vi "Slow Axis Waveform Generator.vi"(4 "Flyback Lines":u16, 5 "Number Data of Points":i32, 6 "Scan Parameters":T1, 7 "Image Acquisition Parameters":T2={"Scan Type"=enum."Sample Scanning", "Scan Mode"=enum."XY", "Fast Axis Frequency (Hz)"=100.0, "Image Format"=128, "Line Accumulations"=1, "Frames Per Capture"=1, "Frames Accumulations"=1, "Image Dimension (um)"=[], "Number of Z Steps"=1, "Z Steps Size (um)"=1.0, "Pixel Size (nm)"=[]} {"Z Steps Size (um)" min=0.0; "Number of Z Steps" min=1; "Frames Accumulations" min=1; "Frames Per Capture" min=1; "Line Accumulations" min=1; "Image Format" items=["64 x 64"=64, "128 x 128"=128, "256 x 256"=256, "512 x 512"=512, "1024 x 1024"=1024, "2048 x 2048"=2048]}) -> (0 "Linear Ramp End":u32, 1 "Slow Axis Frequency":dbl, 2 "Slow Axis Waveform":dbl[](array[numeric]), 3 "Flyback Lines":u16)   [LabVIEW 2016]
uses:
  Type Defs/Image Acquisition Parameters.ctl
  Scan Parameters.ctl
panel:
  out "XY Graph":cluster{"y":dbl[], "t":dbl[]}(graph)
  # "Copyright (C) 2020 Edward S Allgeyer\n\nRedistribution and use in source and binary forms, with or without\nmodification, are permitted provided that the following conditions\nare met:\n\n1. Redistributions of source code must retain the above copyright\n   notice, this list of conditions and the following disclaimer.\n\n2. Redistributions in binary form must reproduce the above copyright\n   notice, this list of conditions and the following disclaimer in\n   the documentation and/or other materials provided with the\n   distribution.\n\n3. Neither the name of the copyright holder nor the names of its\n   contributors may be used to endorse or promote products derived\n   from this software without specific prior written permission.\n\nTHIS SOFTWARE IS PROVIDED BY THE COPYRIGHT HOLDERS AND CONTRIBUTORS\n\"AS IS\" AND ANY EXPRESS OR IMPLIED WARRANTIES, INCLUDING, BUT NOT\nLIMITED TO, THE IMPLIED WARRANTIES OF MERCHANTABILITY AND FITNESS\nFOR A PARTICULAR PURPOSE ARE DISCLAIMED. IN NO EVENT SHALL THE\nCOPYRIGHT HOLDER OR CONTRIBUTORS BE LIABLE FOR ANY DIRECT, INDIRECT,\nINCIDENTAL, SPECIAL, EXEMPLARY, OR CONSEQUENTIAL DAMAGES (INCLUDING,\nBUT NOT LIMITED TO, PROCUREMENT OF SUBSTITUTE GOODS OR SERVICES;\nLOSS OF USE, DATA, OR PROFITS; OR BUSINESS INTERRUPTION) HOWEVER\nCAUSED AND ON ANY THEORY OF LIABILITY, WHETHER IN CONTRACT, STRICT\nLIABILITY, OR TORT (INCLUDING NEGLIGENCE OR OTHERWISE) ARISING IN\nANY WAY OUT OF THE USE OF THIS SOFTWARE, EVEN IF ADVISED OF THE\nPOSSIBILITY OF SUCH DAMAGE."
  # "XY"
  # "Z"
  # "Length"
  # "Height"
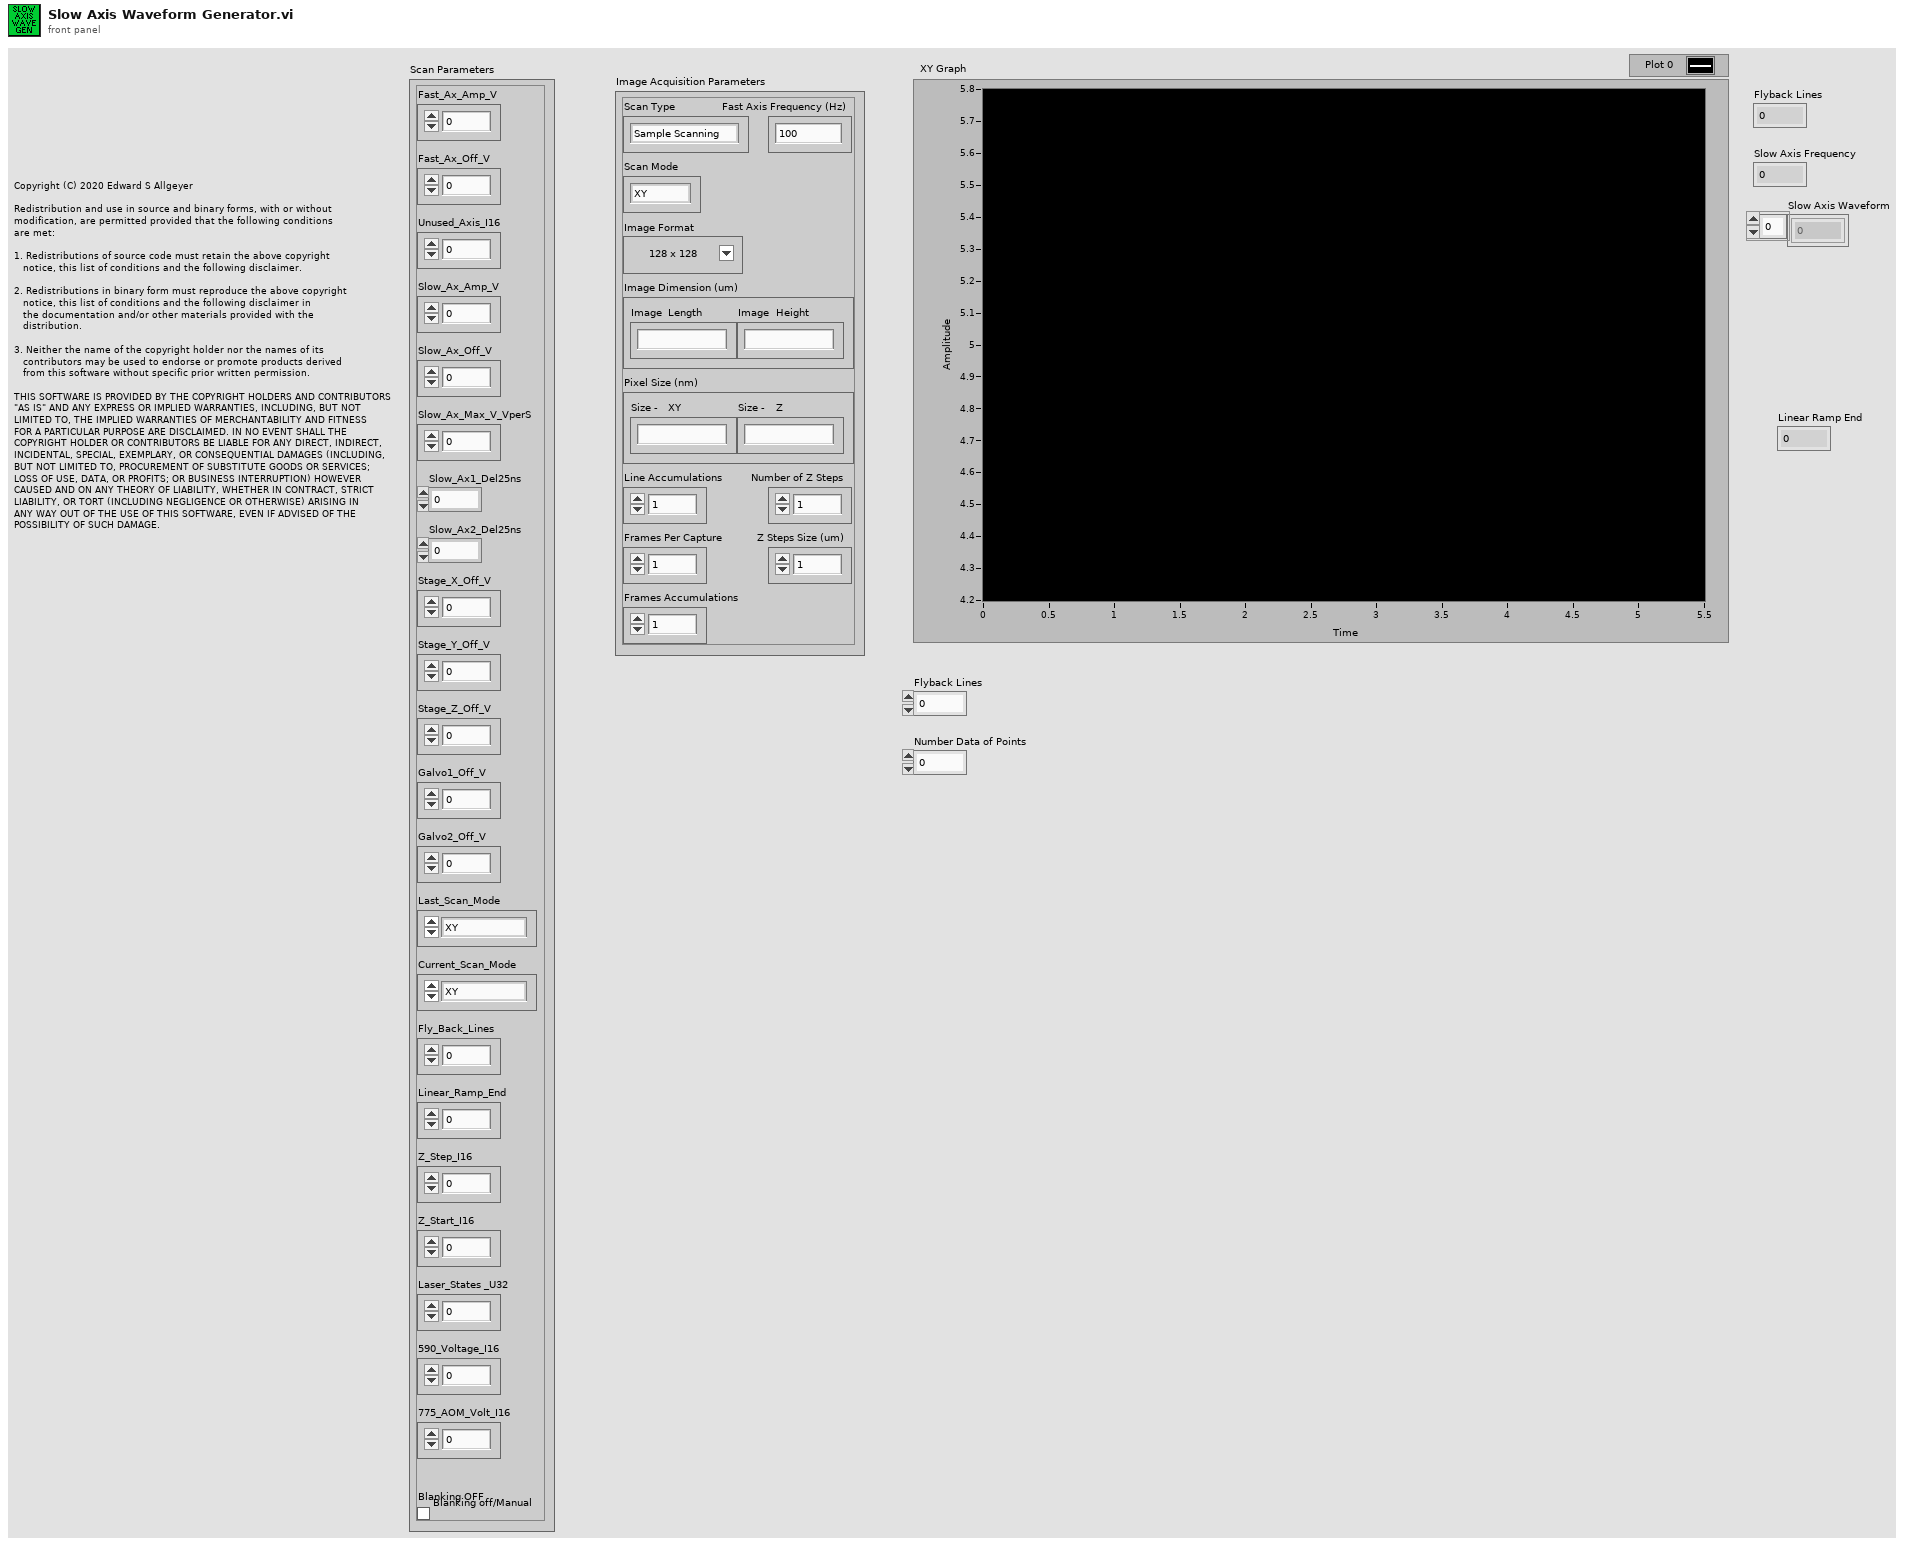
[diagram p1: front panel]
types:
  T1 = typedef "Scan Parameters.ctl" = cluster{"Fast_Ax_Amp_V":dbl, "Fast_Ax_Off_V":dbl, "Slow_Ax_Amp_V":dbl, "Slow_Ax_Off_V ":dbl, "Slow_Ax_Max_V_VperS":dbl, "Slow_Ax1_Del25ns":i32, "Slow_Ax2_Del25ns":i32, "Stage_X_Off_V":dbl, "Stage_Y_Off_V":dbl, "Stage_Z_Off_V":dbl, "Galvo1_Off_V":dbl, "Galvo2_Off_V":dbl, "Last_Scan_Mode":enum16{"XY", "XZ", "YZ", "XYZ"}, "Current_Scan_Mode":enum16{"XY", "XZ", "YZ", "XYZ"}, "Fly_Back_Lines":u16, "Linear_Ramp_End":u32, "Z_Step_I16":i16, "Z_Start_I16":i16, "Laser_States _U32":u32, "590_Voltage_I16":i16, "775_AOM_Volt_I16":i16, "Blanking OFF":bool, "Unused_Axis_I16":i16}
  T2 = typedef "Image Acquisition Parameters.ctl" = cluster{"Scan Type":enum16{"Sample Scanning", "Beam Scanning"}, "Scan Mode":enum16{"XY", "XZ", "YZ", "XYZ"}, "Fast Axis Frequency (Hz)":dbl, "Image Format":u16, "Line Accumulations":u16, "Frames Per Capture":u16, "Frames Accumulations":u16, "Image Dimension (um)":dbl[], "Number of Z Steps":u8, "Z Steps Size (um)":dbl, "Pixel Size (nm)":dbl[]}
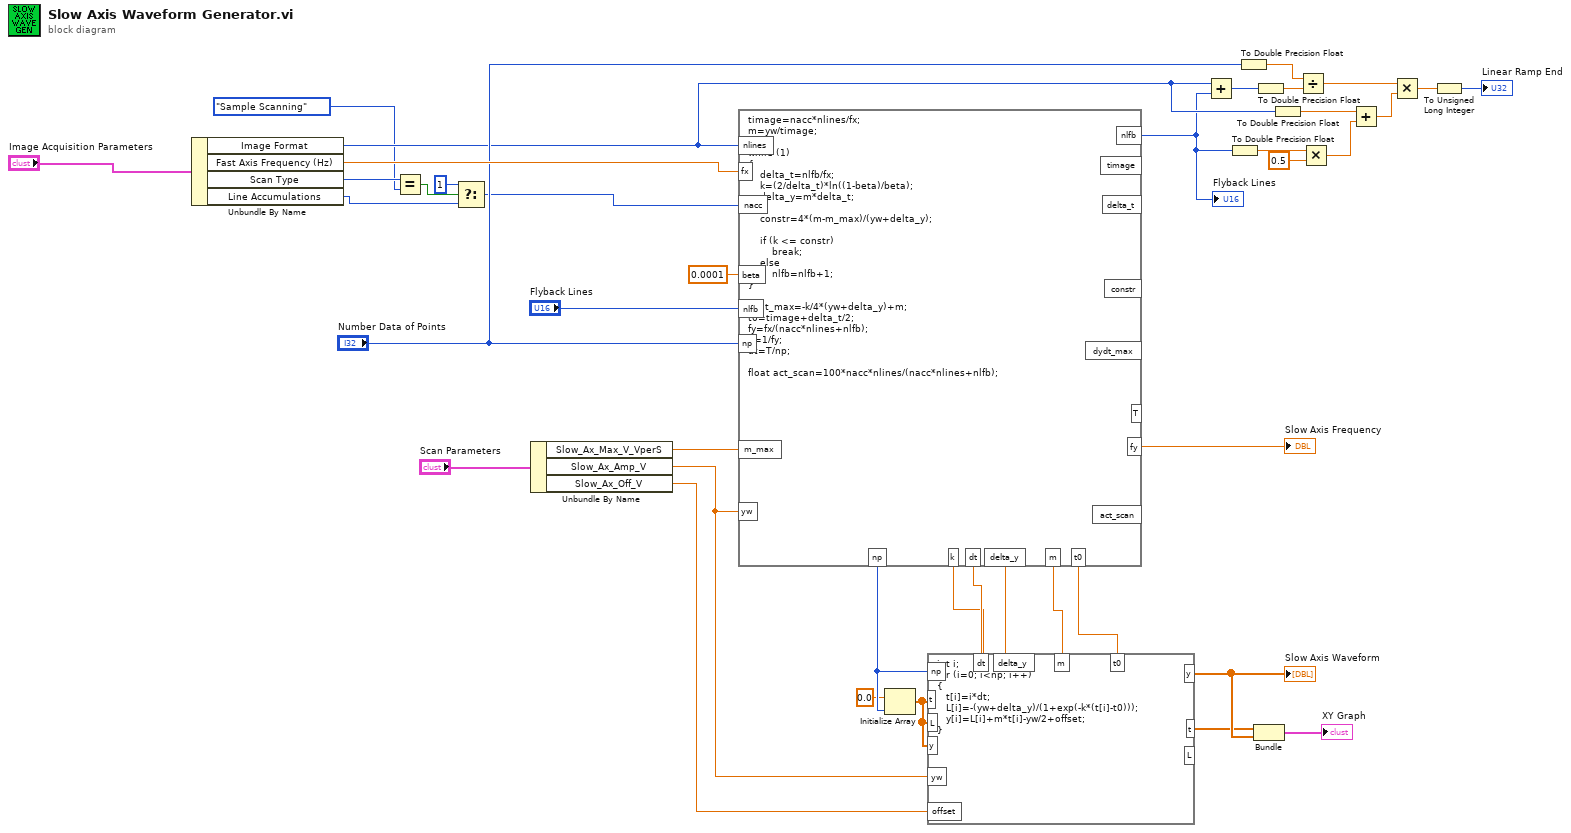
[diagram p0: block diagram]
diagram:
  n1 = Unbundle By Name("Image Acquisition Parameters") -> ("Image Format"=w16:u16, "Fast Axis Frequency (Hz)"=w29:dbl, "Scan Type"=w6:enum16{"Sample Scanning", "Beam Scanning"}, "Line Accumulations"=w3:u16)
  n2 = Equal?(x=w6, y=enum16{"Sample Scanning", "Beam Scanning"}."Sample Scanning") -> (x = y?=w4:bool)
  n3 = Select(t=u16 1, s=w4, f=w3) -> (s? t:f=w1:u16)
  n4 = Unbundle By Name("Scan Parameters") -> ("Slow_Ax_Max_V_VperS"=w25:dbl, "Slow_Ax_Amp_V"=w27:dbl, "Slow_Ax_Off_V"=w26:dbl)
  n5 = formula code="timage=nacc*nlines/fx;\nm=yw/timage; \n\nwhile (1)\n{\n    delta_t=nlfb/fx;\n    k=(2/delta_t)*ln((1-beta)/beta);\n    delta_y=m*delta_t;\n    \n    constr=4*(m-m_max)/(yw+delta_y);\n\n    if (k <= constr)\n        break;\n    else\n        nlfb=nlfb+1;\n}\n\ndydt_max=-k/4*(yw+delta_y)+m;\nt0=timage+delta_t/2;\nfy=fx/(nacc*nlines+nlfb);\nT=1/fy;\ndt=T/np;\n\nfloat act_scan=100*nacc*nlines/(nacc*nlines+nlfb);"("yw"=w27, "fx"=w29, "nlines"=w16, "m_max"=w25, "beta"=0.0001 ("input variable"), "nlfb"="Flyback Lines", "nacc"=w1, "np"="Number Data of Points") -> ("k"=w35:dbl, "m"=w37:dbl, "delta_y"=w36:dbl, "nlfb"=w14:u16, "t0"=w39:dbl, "fy"=→"Slow Axis Frequency":dbl, "dt"=w38:dbl, "np"=w34:i32)  [unwired: 6 out]
  "Flyback Lines" <- w14
  n6 = Initialize Array(0.0 ("element"), w34) -> (w33:dbl[])
  n7 = formula code="int i;\nfor (i=0; i<np; i++)\n{\n   t[i]=i*dt;\n   L[i]=-(yw+delta_y)/(1+exp(-k*(t[i]-t0)));\n   y[i]=L[i]+m*t[i]-yw/2+offset;\n}"("np"=w34, "t"=w33, "L"=w33, "y"=w33, "offset"=w26, "k"=w35, "dt"=w38, "yw"=w27, "delta_y"=w36, "m"=w37, "t0"=w39) -> ("t"=w21:dbl[], "y"=w22:dbl[])  [unwired: 1 out]
  "Slow Axis Waveform" <- w22
  n8 = Add(x=w16, y=w14) -> (x+y=w20:u16)
  n9 = To Double Precision Float(number=w14) -> (double precision float=w12:dbl)
  n10 = To Double Precision Float(number="Number Data of Points") -> (double precision float=w18:dbl)
  n11 = Bundle("t"=w21, "y"=w22) -> (→"XY Graph":cluster{"t":dbl[], "y":dbl[]})  [unwired: 1 in]
  n12 = To Double Precision Float(number=w20) -> (double precision float=w17:dbl)
  n13 = To Double Precision Float(number=w16) -> (double precision float=w10:dbl)
  n14 = Divide(x=w18, y=w17) -> (x/y=w15:dbl)
  n15 = Multiply(x=w12, y=0.5) -> (x*y=w9:dbl)
  n16 = Add(x=w10, y=w9) -> (x+y=w8:dbl)
  n17 = Multiply(x=w15, y=w8) -> (x*y=w11:dbl)
  n18 = To Unsigned Long Integer(number=w11) -> (unsigned 32bit integer=→"Linear Ramp End":u32)
